vi "Open SMO.vi"(8 "error in (no error)":errorcluster, 11 "Instrument in":refnum<class "Instrument.lvclass">) -> (0 "error out":errorcluster, 3 "Instrument out":refnum<class "Instrument.lvclass">)   [LabVIEW 2019, in "Instrument.lvclass"]
uses:
  Instrument.lvclass
  Instrument.lvclass/Instrument.ctl
  RemoteControl/RemoteControl.lvclass
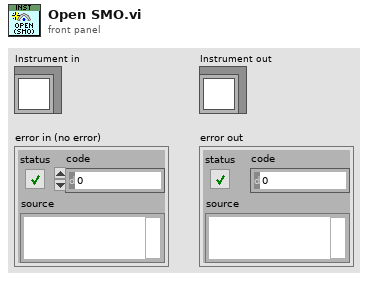
[diagram p1: front panel]
types:
  T1 = typedef "RemoteControl.lvclass/RC Com Type--enum.ctl" = enum16{"RC", "STM", "ZMQ"}
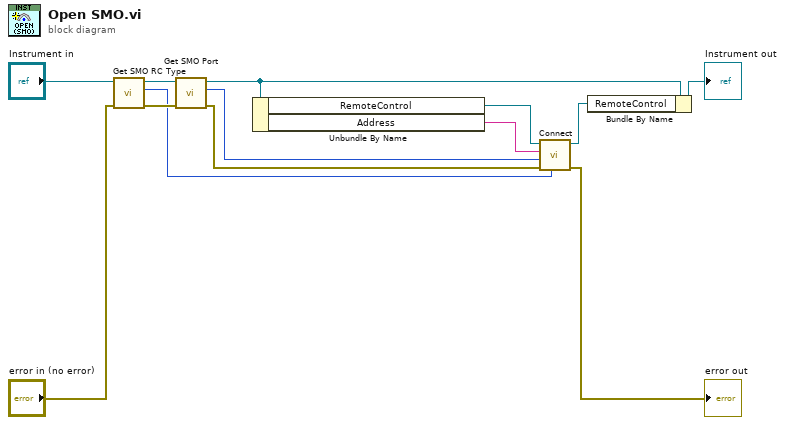
[diagram p0: block diagram]
diagram:
  n1 = call-dynamic "Get SMO RC Type.vi"("error in (no error)"="error in (no error)", "Instrument in"="Instrument in") -> ("error out"=w5:errorcluster, "RC Type"=w2:T1, "Instrument out"=w4:refnum<class "Instrument.lvclass">)  [unwired: 7 in]
  n2 = call-dynamic "Get SMO Port.vi"("error in (no error)"=w5, "Instrument in"=w4) -> ("error out"=w13:errorcluster, "Port"=w3:u16, "Instrument out"=w12:refnum<class "Instrument.lvclass">)  [unwired: 7 in]
  n3 = Unbundle By Name(w12) -> ("RemoteControl"=w8:refnum<class "RemoteControl.lvclass">, "Address"=w1:string)
  n4 = call "Connect.vi"("RC Type"=w2, "error in (no error)"=w13, "Port"=w3, "address"=w1, "RemoteControl in"=w8) -> ("error out"=→"error out":errorcluster, "RemoteControl out"=w9:refnum<class "RemoteControl.lvclass">)  [unwired: 5 in]
  n5 = Bundle By Name(cluster=w12, "RemoteControl"=w9) -> (→"Instrument out":refnum<class "Instrument.lvclass">)
